vi "m10.wfg.vi"(1 "Param 0":dbl=1000.0, 2 "Param 1":dbl, 3 "Param 2":dbl, 4 "Param 3":dbl, 5 "error in (no error)":errorcluster, 8 "Waveform Properties":T1={"Fs (Hz)"=20000.0, "Amplitude (V)"=5.0, "Ramp (s)"=0.02} {"Ramp (s)" min=0.0; "Fs (Hz)" min=0.0}, 10 "Duration (s)":dbl=0.1) -> (14 "Waveform Out":waveform(dbl), 19 "error out":errorcluster)   [LabVIEW 2013]
panel:
  in  "Stimulus Type":u16(ring) items=["Off", "DC", "Noise", "PT", "FM"]
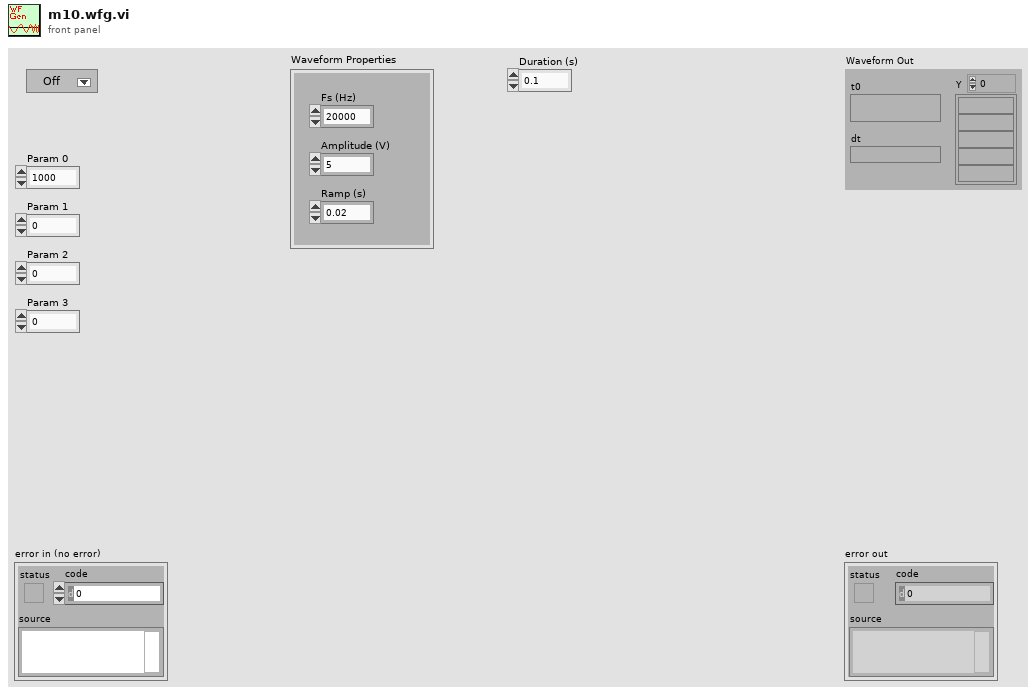
[diagram p1: front panel]
types:
  T1 = cluster{"Fs (Hz)":dbl, "Amplitude (V)":dbl, "Ramp (s)":dbl}
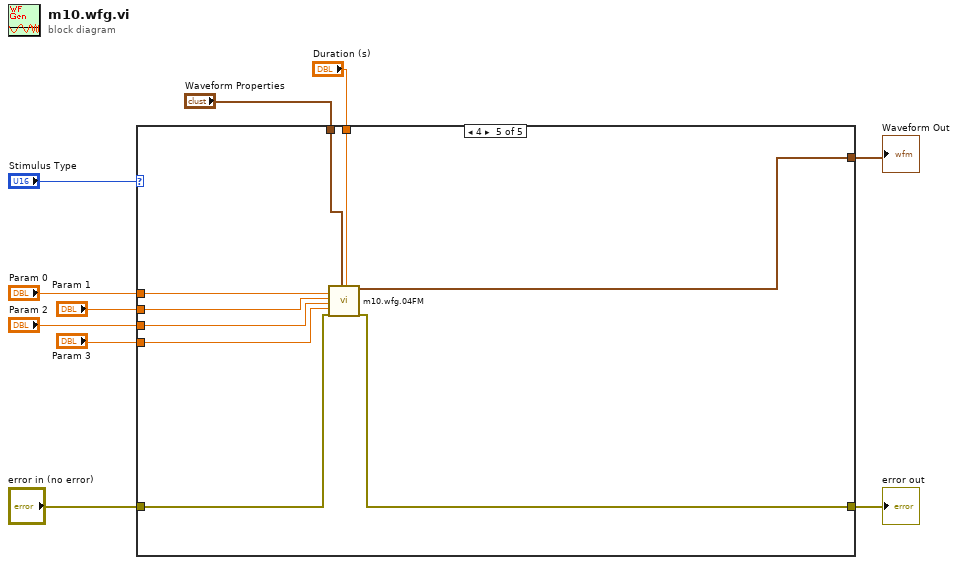
[diagram p0: block diagram]
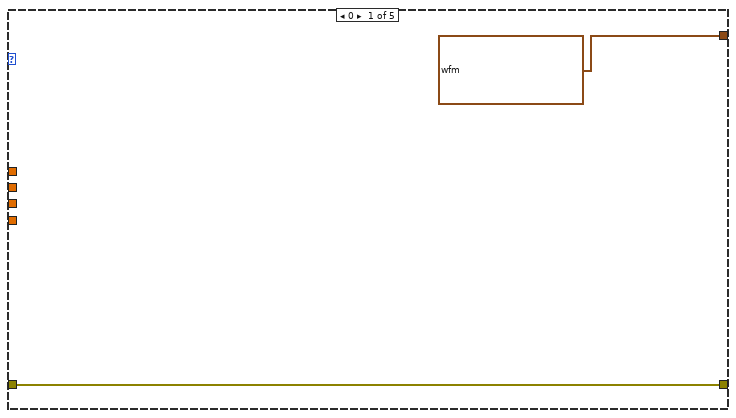
[diagram p2: hidden frame]
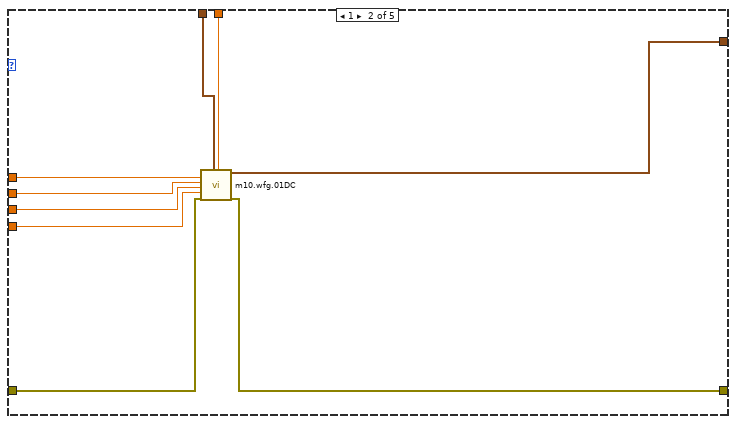
[diagram p3: hidden frame]
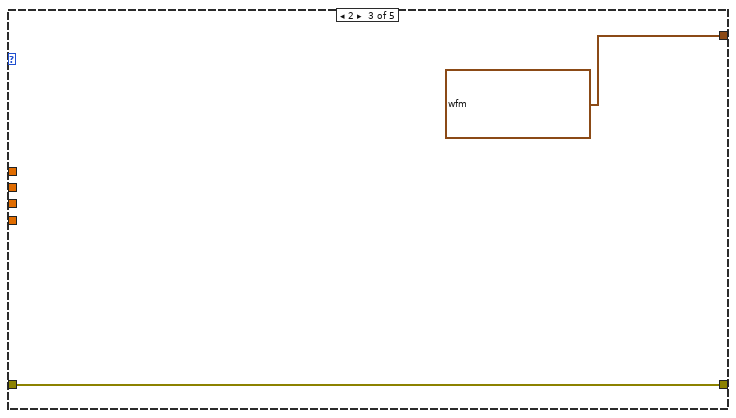
[diagram p4: hidden frame]
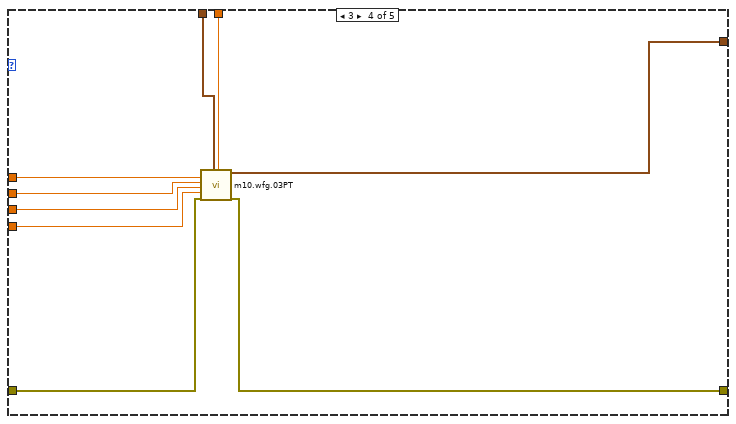
[diagram p5: hidden frame]
diagram:
  n1 = case shown="4" "Stimulus Type" {
    tunnel: "Param 0" -> [_ w21 _ w32 w41]
    tunnel: "Param 1" -> [_ w20 _ w31 w40]
    tunnel: "Param 2" -> [_ w19 _ w30 w39]
    tunnel: "Param 3" -> [_ w18 _ w29 w38]
    tunnel: "Waveform Properties" -> [_ w17 _ w28 w37]
    tunnel: "Duration (s)" -> [_ w16 _ w27 w36]
    tunnel: "error in (no error)" -> [w11 w15 w23 w26 w35]
    tunnel: [w11 w14 w23 w25 w34] -> w2
    tunnel: [waveform(dbl) {"t0"=timestamp(0 s since 1904-01-01), "dt"=1.0, "Y"=[]} ("Waveform") w13 waveform(dbl) {"t0"=timestamp(0 s since 1904-01-01), "dt"=1.0, "Y"=[]} ("Waveform") w24 w33] -> w1
    frame 0 {
    }
    frame 1 {
      n2 = call "m10.wfg.01DC.vi"("Param 0"=w21, "Param 1"=w20, "Param 2"=w19, "Param 3"=w18, "error in (no error)"=w15, "Waveform Properties"=w17, "Duration (s)"=w16) -> ("Waveform Out"=w13:waveform(dbl), "error out"=w14:errorcluster)  [unwired: 11 in]
    }
    frame 2 {
    }
    frame 3 {
      n3 = call "m10.wfg.03PT.vi"("Param 0"=w32, "Param 1"=w31, "Param 2"=w30, "Param 3"=w29, "error in (no error)"=w26, "Waveform Properties"=w28, "Duration (s)"=w27) -> ("Waveform Out"=w24:waveform(dbl), "error out"=w25:errorcluster)  [unwired: 11 in]
    }
    frame 4 {
      n4 = call "m10.wfg.04FM.vi"("Param 0"=w41, "Param 1"=w40, "Param 2"=w39, "Param 3"=w38, "error in (no error)"=w35, "Waveform Properties"=w37, "Duration (s)"=w36) -> ("Waveform Out"=w33:waveform(dbl), "error out"=w34:errorcluster)  [unwired: 11 in]
    }
  }
  "Waveform Out" <- w1
  "error out" <- w2
